vi "Frames.Export.vi"(8 "error in (no error)":errorcluster, 10 "GUID":string, 11 "Item Ref in":T4 format="%.0x") -> (0 "error out":errorcluster, 2 "Section":T1 {"Frames"."Signals"."Byte Order" items=["Little Endian", "Big Endian"]; "Frames"."Signals"."Data Type" items=["Signed", "Unsigned", "IEEE Float"]}, 3 "Section Ref out":T4 format="%.0x")   [LabVIEW 2015, in "Diagnostics Addon System Explorer.lvlib"]
uses:
  Diagnostics Addon System Explorer.lvlib
  <vilib>/NI Veristand/Custom Device API/Custom Device Item Ref.ctl
  Types/Frames.Export.ctl
  Types/Frame.Export.ctl
  Shared/Types/Signal.ctl
  ID.FG.vi
  Get Signals.vi
  Type.FG.vi
  Signal.FG.vi
  <vilib>/NI Veristand/Custom Device API/NI VeriStand - Get Custom Device Channel Data.vi
  <vilib>/NI Veristand/Custom Device API/NI VeriStand - Get Item Property.vi
  <vilib>/NI Veristand/Custom Device API/Get Item Property (String).vi
  <vilib>/NI Veristand/Custom Device API/Get Item Property (Double).vi
  <vilib>/NI Veristand/Custom Device API/Get Item Property (U32).vi
  <vilib>/NI Veristand/Custom Device API/NI VeriStand - Set Item Property.vi
  <vilib>/NI Veristand/Custom Device API/Set Item Property (String).vi
  <vilib>/NI Veristand/Custom Device API/Set Item Property (Double).vi
  <vilib>/NI Veristand/Custom Device API/Set Item Property (U32).vi
  Shared/SubVIs/GUID Lookup.vi
  <vilib>/NI Veristand/Custom Device API/NI VeriStand - Get Item Data.vi
  <vilib>/NI Veristand/Custom Device Tools/Custom Device Utility Library/NI VeriStand - Search for Item by GUID.vi
  <vilib>/NI Veristand/Custom Device Tools/Custom Device Utility Library/Custom Device Utility Library.lvlib
  <vilib>/NI Veristand/Custom Device API/Custom Device API.lvlib
  Shared/Diagnostics Addon Shared.lvlib
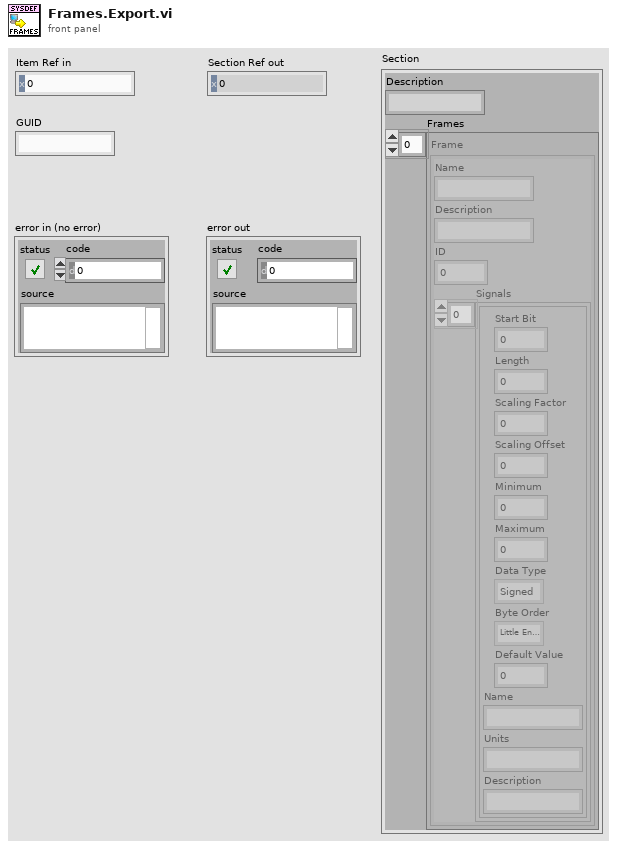
[diagram p1: front panel]
types:
  T1 = typedef "Diagnostics Addon System Explorer.lvlib/Frames.Export.ctl" = cluster{"Description":string, "Frames":T2[]}
  T2 = typedef "Diagnostics Addon System Explorer.lvlib/Frame.Export.ctl" = cluster{"Name":string, "Description":string, "ID":u32, "Signals":T3[]}
  T3 = typedef "Diagnostics Addon Shared.lvlib/Signal.ctl" = cluster{"Start Bit":u8, "Length":u8, "Scaling Factor":dbl, "Scaling Offset":dbl, "Minimum":dbl, "Maximum":dbl, "Data Type":u32, "Byte Order":u32, "Default Value":dbl, "Name":string, "Units":string, "Description":string}
  T4 = typedef "Custom Device API.lvlib/Custom Device Item Ref.ctl" = u64
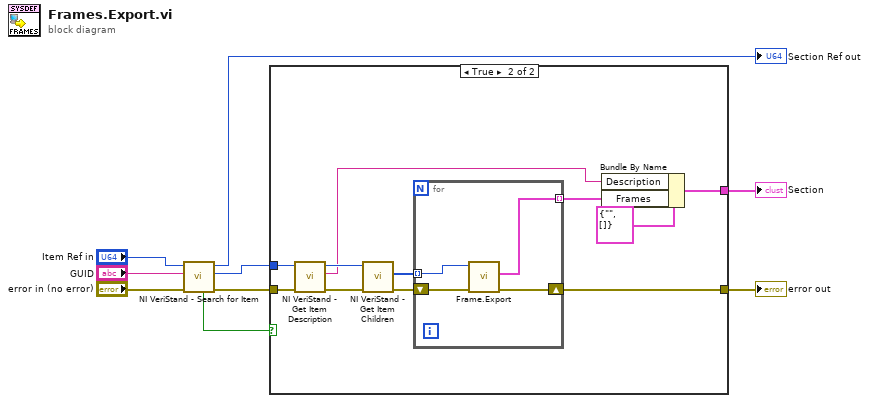
[diagram p0: block diagram]
diagram:
  n1 = call-poly <vilib>:"NI VeriStand - Search for Item.vi"("error in"="error in (no error)", "Item GUID"="GUID", "Section Ref in"="Item Ref in") -> ("error out"=w4:errorcluster, "Item Ref"=w3:T4, "Section Ref out"=→"Section Ref out":T4, "Found"=w2:bool)  [unwired: 5 in]
  n2 = case shown="True" w2 {
    tunnel: [_ w12] -> w1
    tunnel: [w10 w21] -> w5
    tunnel: w4 -> [w10 w16]
    tunnel: w3 -> [_ w18]
    frame False {
    }
    frame True {
      n3 = call <vilib>:"NI VeriStand - Get Item Description.vi"("error in (no error)"=w16, "Item Ref in"=w18) -> ("error out"=w15:errorcluster, "Description"=w13:string, "Item Ref out"=w17:T4)  [unwired: 7 out]
      n4 = call <vilib>:"NI VeriStand - Get Item Children.vi"("error in (no error)"=w15, "Item Ref in"=w17) -> ("error out"=w20:errorcluster, "Child Refs"=w19:T4[])  [unwired: 6 in, 2 out]
      n5 = for {
        tunnel: w19 -> [w22] mode=indexing
        shift-right: [w23] -> w21
        shift-left: w20 -> [w24]
        tunnel: [w25] -> w11 mode=indexing
        n6 = call "Frame.Export.vi"("error in (no error)"=w24, "Item Ref in"=w22) -> ("error out"=w23:errorcluster, "Frame"=w25:T2)  [unwired: 7 in, 1 out]
      }
      n7 = Bundle By Name(cluster=T1 {"Description"="", "Frames"=[]}, "Description"=w13, "Frames"=w11) -> (w12:T1)
    }
  }
  "error out" <- w5
  "Section" <- w1
